vi "GetSetCommStatus.vi"(8 "error in":errorcluster, 9 "Coded integer comm status":i32 min=0 max=255 step=1, 10 "get/set":T1=enum."set", 11 "VISA resource name":refnum<visa-resource-name>) -> (0 "error out":errorcluster, 1 "Comm status Value":i32, 2 "Comm status String Value":string, 3 "VISA resource name out":refnum<visa-resource-name>)   [LabVIEW 2023, in "Thermotron 8800.lvlib"]
doc: "CMST\nCommand name: Comm status\nCommand type: System status\nDescription: This query command asks the 8800 for the current comm status. The 8800 sends a\ncoded integer value. The edit operation command changes the current comm status.\nThe CMST data byte is defined as follows:\nBits 0 – 7\n1 = Send acknowledge\n2, 4, 8, 16, 32, 64, 128 = unused\nSyntax: CMST? or CMSTn\nWhere n is the new comm status.\nData type: Coded integer\nQuery example: CMST?\n8800 response: 1 (send acknowledge is on)\nOperation example: CMST0\n8800 response: The 8800 turns off send acknowledge."
uses:
  Thermotron 8800.lvlib
  Private/get set.ctl
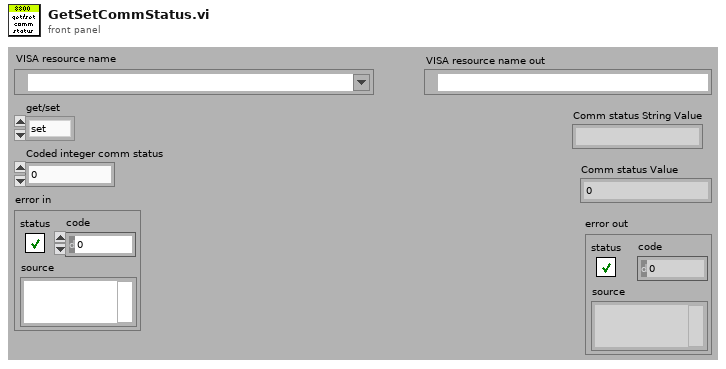
[diagram p1: front panel]
types:
  T1 = typedef "Thermotron 8800.lvlib/get set.ctl" = enum16{"get", "set"}
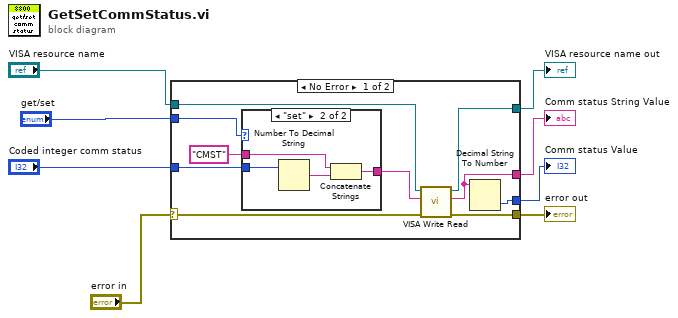
[diagram p0: block diagram]
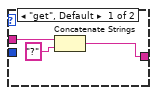
[diagram p2: hidden frame]
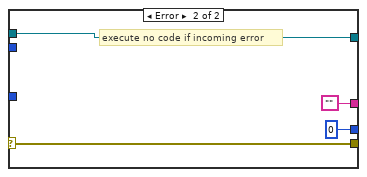
[diagram p3: hidden frame]
diagram:
  n1 = case shown="No Error" "error in" {
    selector: "error in" -> [w9 w28]
    tunnel: "get/set" -> [w18 _]
    tunnel: [w15 ""] -> w7
    tunnel: [w14 0] -> w6
    tunnel: [w13 w28] -> w5
    tunnel: [w12 w29] -> w4
    tunnel: "VISA resource name" -> [w11 w29]
    tunnel: "Coded integer comm status" -> [w10 _]
    frame No Error {
      n2 = case shown="\"set\"" w18 {
        tunnel: "CMST" ("8800 Command") -> [w20 w25]
        tunnel: [w21 w24] -> w16
        tunnel: w10 -> [_ w22]
        frame "get", Default {
          n3 = Concatenate Strings(w20, "?" ("8800 Command")) -> (w21:string)
        }
        frame "set" {
          n4 = Number To Decimal String(number=w22) -> (decimal integer string=w23:string)  [unwired: 1 in]
          n5 = Concatenate Strings(w25, w23) -> (w24:string)
        }
      }
      n6 = call "VISA Write Read.vi"("error in (no error)"=w9, "8800 Command"=w16, "VISA Refnum in"=w11) -> ("error out"=w13:errorcluster, "read buffer"=w15:string, "VISA Refnum out"=w12:refnum<visa-resource-name>)  [unwired: 6 in]
      n7 = Decimal String To Number(string=w15) -> (number=w14:i32)  [unwired: 2 in, 1 out]
    }
    frame Error {
      # "execute no code if incoming error"
    }
  }
  "VISA resource name out" <- w4
  "error out" <- w5
  "Comm status String Value" <- w7
  "Comm status Value" <- w6
